vi "Key Pressed.vi"(8 "error in (no error)":errorcluster, 10 "Key Pressed":i32, 11 "Keypad in":refnum<class "Keypad.lvclass">) -> (0 "error out":errorcluster, 3 "Keypad out":refnum<class "Keypad.lvclass">)   [LabVIEW 2020, in "Keypad.lvlib" / "Keypad.lvclass"]
uses:
  Keypad.lvclass
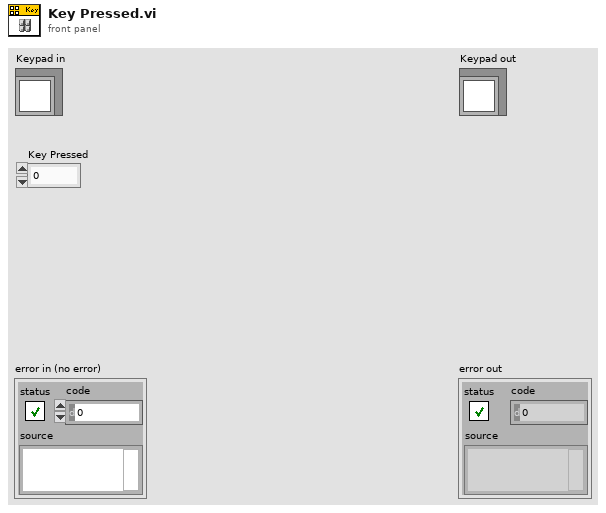
[diagram p1: front panel]
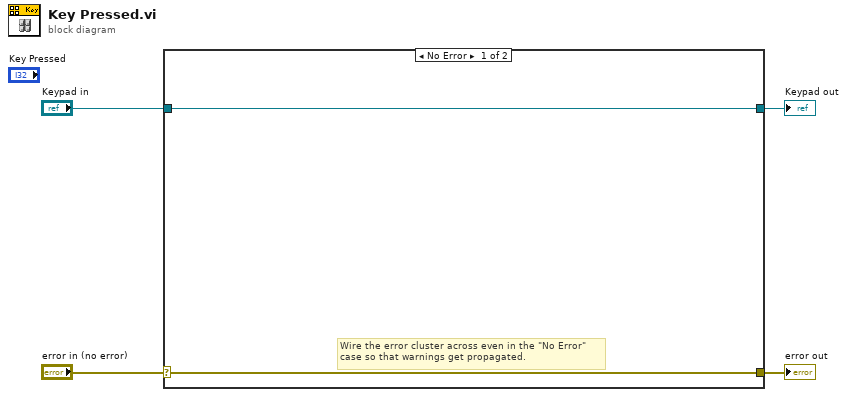
[diagram p0: block diagram]
diagram:
  n1 = case shown="No Error" "error in (no error)" {
    selector: "error in (no error)" -> [w5 w8]
    tunnel: [w5 w8] -> w3
    tunnel: [w6 w7] -> w1
    tunnel: "Keypad in" -> [w6 w7]
    frame No Error {
      # "Wire the error cluster across even in the \"No Error\"\ncase so that warnings get propagated."
    }
    frame Error {
    }
  }
  "error out" <- w3
  "Keypad out" <- w1
